vi "Initialize TCP Refs.vi"(8 "error in (no error)":errorcluster, 11 "Name":string) -> (0 "error out":errorcluster, 3 "TCP Refs":T1)   [LabVIEW 2015, in "Diagnostics Addon Engine.lvlib"]
uses:
  Diagnostics Addon Engine.lvlib
  Types/TCP Refs.ctl
  STM/STM Lookup Table Ref.ctl
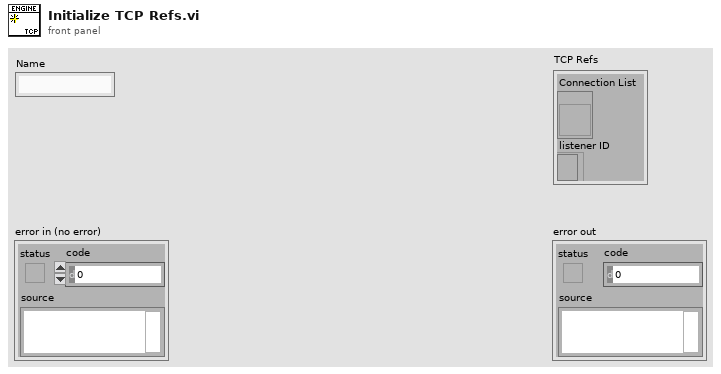
[diagram p1: front panel]
types:
  T1 = typedef "Diagnostics Addon Engine.lvlib/TCP Refs.ctl" = cluster{"Connection List":T2, "listener ID":refnum<k5>}
  T2 = typedef "Diagnostics Addon Engine.lvlib/STM Lookup Table Ref.ctl" = refnum<vi>
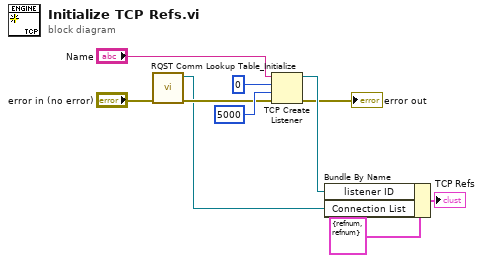
[diagram p0: block diagram]
diagram:
  n1 = call "RQST Comm Lookup Table_Initialize.vi"("error in (no error)"="error in (no error)") -> ("error out"=w6:errorcluster, "vi reference"=w2:T2)  [unwired: 9 in]
  n2 = TCP Create Listener(8:w6, 9:5000 ("timeout ms (25000)"), 10:u16 0 ("port"), 11:"Name") -> (0:→"error out":errorcluster, 3:w9:refnum<k5>)  [unwired: 1 in, 1 out]
  n3 = Bundle By Name(cluster=T1 {"Connection List"=refnum, "listener ID"=refnum}, "listener ID"=w9, "Connection List"=w2) -> (→"TCP Refs":T1)
